vi "BK Precision 8600 Series Run Buffer Storage Operation.vi"() -> ()   [LabVIEW 2018]
doc: "Exemplifies how to setup and initiate a buffer storage operation."
uses:
  <instrlib>/BK Precision 8600 Series/BK Precision 8600 Series.lvlib
panel:
  out "Operation Complete":bool
  out "Points Remaining":string
  in  "Trigger Delay (0)":dbl min=0.0 max=3600.0 step=0.01 format="%#.2f"
  in  "Time Interval (1)":dbl=2e-05 min=0.0002 max=3600.0 step=1.0 format="%#_5f"
  in  "Enable Filter (F: False)":bool
  in  "Storage Type (2:All)":u16(ring) items=["Voltage", "Current", "All"]
  in  "Number of Points (2)":dbl=2.0 min=2.0 max=2000.0 step=1.0 format="%#.0f"
  in  "Serial Configuration":cluster{"Baud Rate":u32}={"Baud Rate"=9600} {"Baud Rate" items=["300"=300, "600"=600, "1200"=1200, "2400"=2400, "4800"=4800, "9600"=9600, "19200"=19200]}
  in  "VISA resource name":refnum<visa-resource-name>
  # "(c) 2014-2019 B&K Precision Corporation.  ALL RIGHTS RESERVED."
  # "s"
  # "s"
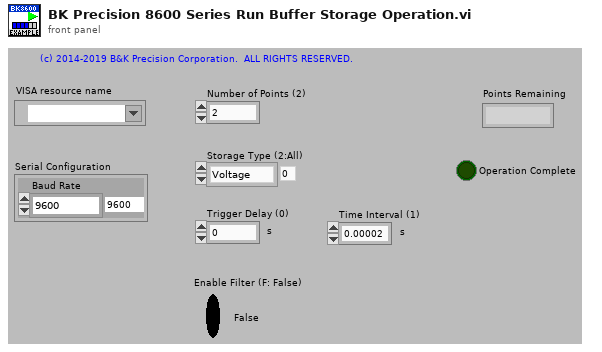
[diagram p1: front panel]
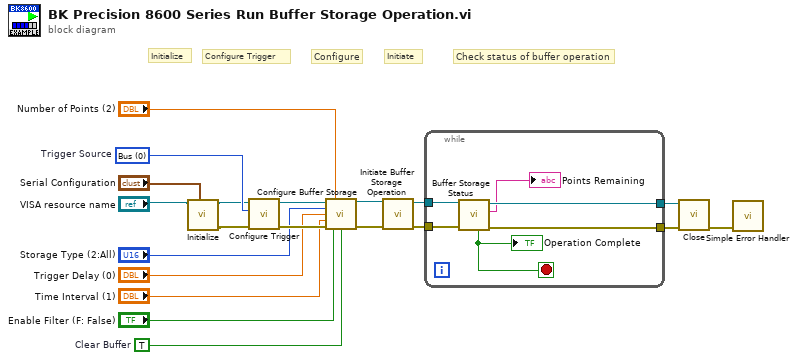
[diagram p0: block diagram]
diagram:
  w5 = u16 0 items=["Bus", "External", "Hold", "Manual", "Timed"]  # Trigger Source
  w9 = TRUE  # Clear Buffer
  # "Check status of buffer operation"
  # "Initiate"
  # "Configure"
  # "Configure Trigger"
  # "Initialize"
  n1 = call <instrlib>:"Initialize.vi"("Serial Configuration"="Serial Configuration", "VISA resource name"="VISA resource name") -> ("error out"=w4:errorcluster, "VISA resource name out"=w3:refnum<visa-resource-name>)  [unwired: 8 in]
  n2 = call <instrlib>:"Configure Trigger.vi"("error in (no error)"=w4, "Trigger Source (0:Bus)"=w5, "VISA resource name"=w3) -> ("error out"=w20:errorcluster, "VISA resource name out"=w19:refnum<visa-resource-name>)  [unwired: 7 in]
  n3 = call <instrlib>:"Configure Buffer Storage.vi"("VISA resource name"=w19, "Number of Points (2)"="Number of Points (2)", "Storage Type (2:All)"="Storage Type (2:All)", "Trigger Delay (0)"="Trigger Delay (0)", "Time Interval (1)"="Time Interval (1)", "error in (no error)"=w20, "Enable Filter (F: False)"="Enable Filter (F: False)", "Clear Buffer? (T: True)"=w9) -> ("VISA resource name out"=w17:refnum<visa-resource-name>, "error out"=w18:errorcluster)  [unwired: 6 in]
  n4 = call <instrlib>:"Initiate Buffer Storage Operation.vi"("error in (no error)"=w18, "VISA resource name"=w17) -> ("error out"=w15:errorcluster, "VISA resource name out"=w16:refnum<visa-resource-name>)  [unwired: 8 in]
  n5 = while {
    tunnel: w16 -> [w26]
    tunnel: w15 -> [w25]
    tunnel: [w24] -> w8
    tunnel: [w23] -> w7
    stop <- w21 stop-if-true
    n6 = call <instrlib>:"Buffer Storage Status.vi"("error in (no error)"=w25, "VISA resource name"=w26) -> ("error out"=w24:errorcluster, "Points Remaining"=→"Points Remaining":string, "VISA resource name out"=w23:refnum<visa-resource-name>, "Operation Complete?"=w21:bool)  [unwired: 5 in, 1 out]
    "Operation Complete" <- w21
  }
  n7 = call <instrlib>:"Close.vi"("error in (no error)"=w8, "VISA resource name"=w7) -> ("error out"=w6:errorcluster)  [unwired: 9 in]
  n8 = call <vilib>:"Simple Error Handler.vi"("error in (no error)"=w6) -> ()  [unwired: 4 in, 5 out]
